vi "20180321.vi"() -> ()   [LabVIEW 2013]
panel:
  in  "Array":void[][](array[numeric])
  in  "stop":bool
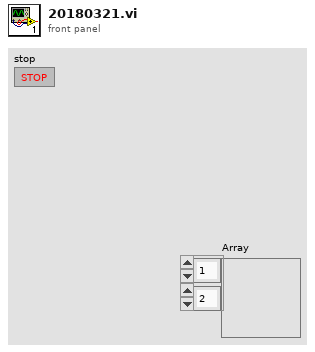
[diagram p1: front panel]
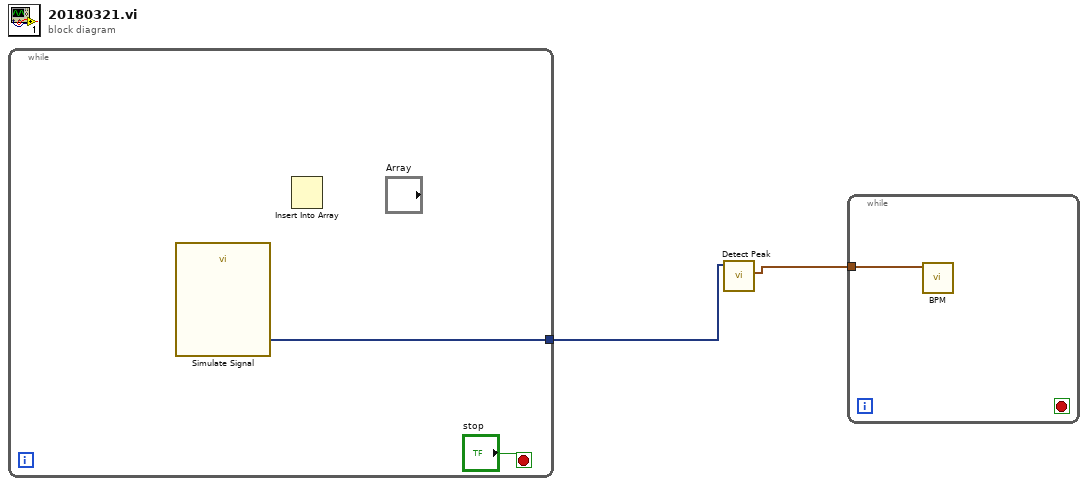
[diagram p0: block diagram]
diagram:
  n1 = while {
    tunnel: [w3] -> w2
    stop <- "stop" stop-if-true
    n2 = call "Simulate Signal"() -> ("Sine"=w3:dynamicdata)  [unwired: 14 in, 1 out]
    n3 = Insert Into Array() -> ()  [unwired: 3 in, 1 out]
  }
  n4 = call "Detect Peak.vi"("Filtered Signal"=w2) -> ("Peak Time Stamp"=w1:timestamp)  [unwired: 7 in, 3 out]
  n5 = while {
    tunnel: w1 -> [w5]
    stop <- _ stop-if-true
    n6 = call "BPM.vi"("Time Stamp"=w5) -> ()  [unwired: 4 in, 3 out]
  }
